vi "Get Core APIs.vi"(8 "error in (no error)":errorcluster, 11 "Task in":refnum<class "Task.lvclass">) -> (0 "error out":errorcluster, 2 "Core APIs":T1, 3 "Task out":refnum<class "Task.lvclass">)   [LabVIEW 2020, in "Volatus.lvlib" / "Task.lvclass"]
uses:
  Task.lvclass
  Core APIs.ctl
  VolatusAPI/VolatusAPI.lvclass
  Event API/EventAPI.lvclass
  Task.lvclass/Task.ctl
  Volatus.lvlib
  TelemetryAPI/TelemetryAPI.lvclass
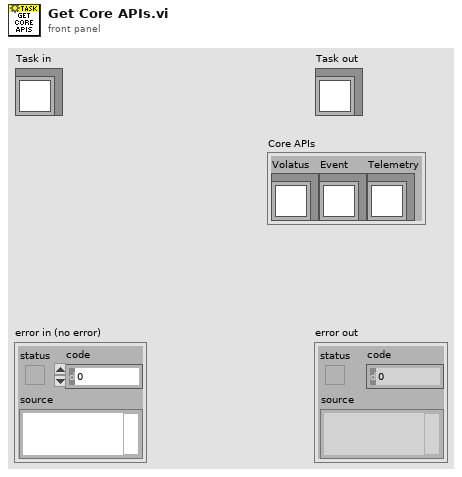
[diagram p1: front panel]
types:
  T1 = typedef "Volatus.lvlib/Core APIs.ctl" = cluster{"Volatus":refnum<class "VolatusAPI.lvclass">, "Event":refnum<class "EventAPI.lvclass">, "Telemetry":refnum<class "TelemetryAPI.lvclass">}
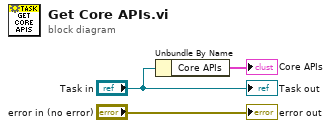
[diagram p0: block diagram]
diagram:
  n1 = Unbundle By Name("Task in") -> ("Core APIs"=→"Core APIs":T1)
  "error out" <- "error in (no error)"
  "Task out" <- "Task in"
